vi "Setup_Scan_Range.vi"(7 "Calling VI Ref":refnum<vi>) -> ()   [LabVIEW 2016]
uses:
  <vilib>/Utility/miscctls.llb/LVPointTypeDef.ctl
  Z Scan Standard Action.ctl
panel:
  in  "Exit":bool
  out "Range (µm)":dbl
  out "Step Size (µm)":dbl
  in  "Number of Steps":u16
  out "End Position (µm)":dbl
  out "Start Position (µm)":dbl
  in  "Set End":bool
  in  "Set Start":bool
  # "Copyright (C) 2020 Edward S Allgeyer\n\nRedistribution and use in source and binary forms, with or without\nmodification, are permitted provided that the following conditions\nare met:\n\n1. Redistributions of source code must retain the above copyright\n   notice, this list of conditions and the following disclaimer.\n\n2. Redistributions in binary form must reproduce the above copyright\n   notice, this list of conditions and the following disclaimer in\n   the documentation and/or other materials provided with the\n   distribution.\n\n3. Neither the name of the copyright holder nor the names of its\n   contributors may be used to endorse or promote products derived\n   from this software without specific prior written permission.\n\nTHIS SOFTWARE IS PROVIDED BY THE COPYRIGHT HOLDERS AND CONTRIBUTORS\n\"AS IS\" AND ANY EXPRESS OR IMPLIED WARRANTIES, INCLUDING, BUT NOT\nLIMITED TO, THE IMPLIED WARRANTIES OF MERCHANTABILITY AND FITNESS\nFOR A PARTICULAR PURPOSE ARE DISCLAIMED. IN NO EVENT SHALL THE\nCOPYRIGHT HOLDER OR CONTRIBUTORS BE LIABLE FOR ANY DIRECT, INDIRECT,\nINCIDENTAL, SPECIAL, EXEMPLARY, OR CONSEQUENTIAL DAMAGES (INCLUDING,\nBUT NOT LIMITED TO, PROCUREMENT OF SUBSTITUTE GOODS OR SERVICES;\nLOSS OF USE, DATA, OR PROFITS; OR BUSINESS INTERRUPTION) HOWEVER\nCAUSED AND ON ANY THEORY OF LIABILITY, WHETHER IN CONTRACT, STRICT\nLIABILITY, OR TORT (INCLUDING NEGLIGENCE OR OTHERWISE) ARISING IN\nANY WAY OUT OF THE USE OF THIS SOFTWARE, EVEN IF ADVISED OF THE\nPOSSIBILITY OF SUCH DAMAGE."
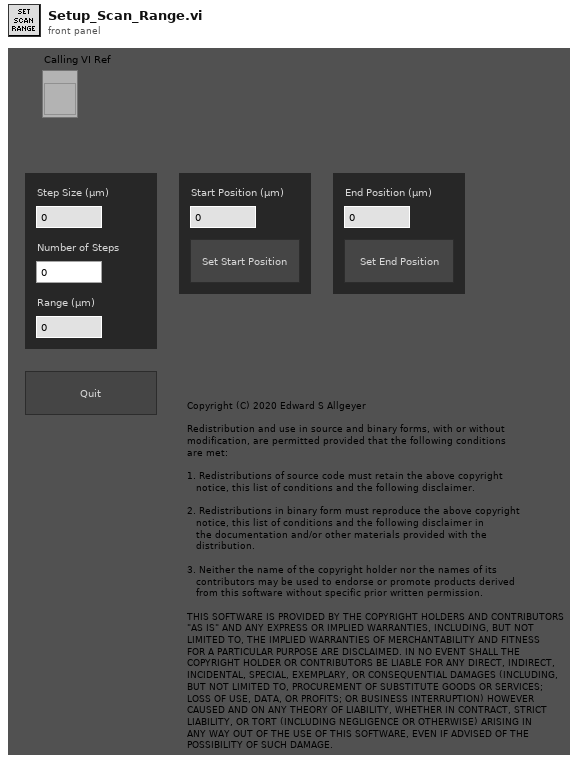
[diagram p1: front panel]
types:
  T1 = enum16{"Always On", "Always Off", "Off While Running"}
  T2 = typedef "LVPointTypeDef.ctl" = cluster{"Horizontal":i16, "Vertical":i16}
  T3 = typedef "Scanning Conversions.ctl" = cluster{"Stage X Axis (Volts/um)":dbl, "Stage Y Axis (Volts/um)":dbl, "Stage Z Axis (Volts/um)":dbl}
  T4 = typedef "Z Scan Standard Action.ctl" = enum16{"Read", "Write"}
  T5 = typedef "Axis Scan Range Parameters.ctl" = cluster{"Start Position (µm)":dbl, "End Position (µm)":dbl, "Step Size (µm)":dbl, "Number of Steps":u16, "Step Direction":bool}
  T6 = typedef "Scan Parameters.ctl" = cluster{"Fast_Ax_Amp_V":dbl, "Fast_Ax_Off_V":dbl, "Slow_Ax_Amp_V":dbl, "Slow_Ax_Off_V ":dbl, "Slow_Ax_Max_V_VperS":dbl, "Slow_Ax1_Del25ns":i32, "Slow_Ax2_Del25ns":i32, "Stage_X_Off_V":dbl, "Stage_Y_Off_V":dbl, "Stage_Z_Off_V":dbl, "Galvo1_Off_V":dbl, "Galvo2_Off_V":dbl, "Last_Scan_Mode":enum16{"XY", "XZ", "YZ", "XYZ"}, "Current_Scan_Mode":enum16{"XY", "XZ", "YZ", "XYZ"}, "Fly_Back_Lines":u16, "Linear_Ramp_End":u32, "Z_Step_I16":i16, "Z_Start_I16":i16, "Laser_States _U32":u32, "590_Voltage_I16":i16, "775_AOM_Volt_I16":i16, "Blanking OFF":bool, "Unused_Axis_I16":i16}
  T7 = typedef "Image Acquisition Parameters.ctl" = cluster{"Scan Type":enum16{"Sample Scanning", "Beam Scanning"}, "Scan Mode":enum16{"XY", "XZ", "YZ", "XYZ"}, "Fast Axis Frequency (Hz)":dbl, "Image Format":u16, "Line Accumulations":u16, "Frames Per Capture":u16, "Frames Accumulations":u16, "Image Dimension (um)":dbl[], "Number of Z Steps":u8, "Z Steps Size (um)":dbl, "Pixel Size (nm)":dbl[]}
  T8 = typedef "LVRectTypeDef.ctl" = cluster{"Left":i16, "Top":i16, "Right":i16, "Bottom":i16}
  T9 = typedef "LVBoundsTypeDef.ctl" = cluster{"Width":u32, "Height":u32}
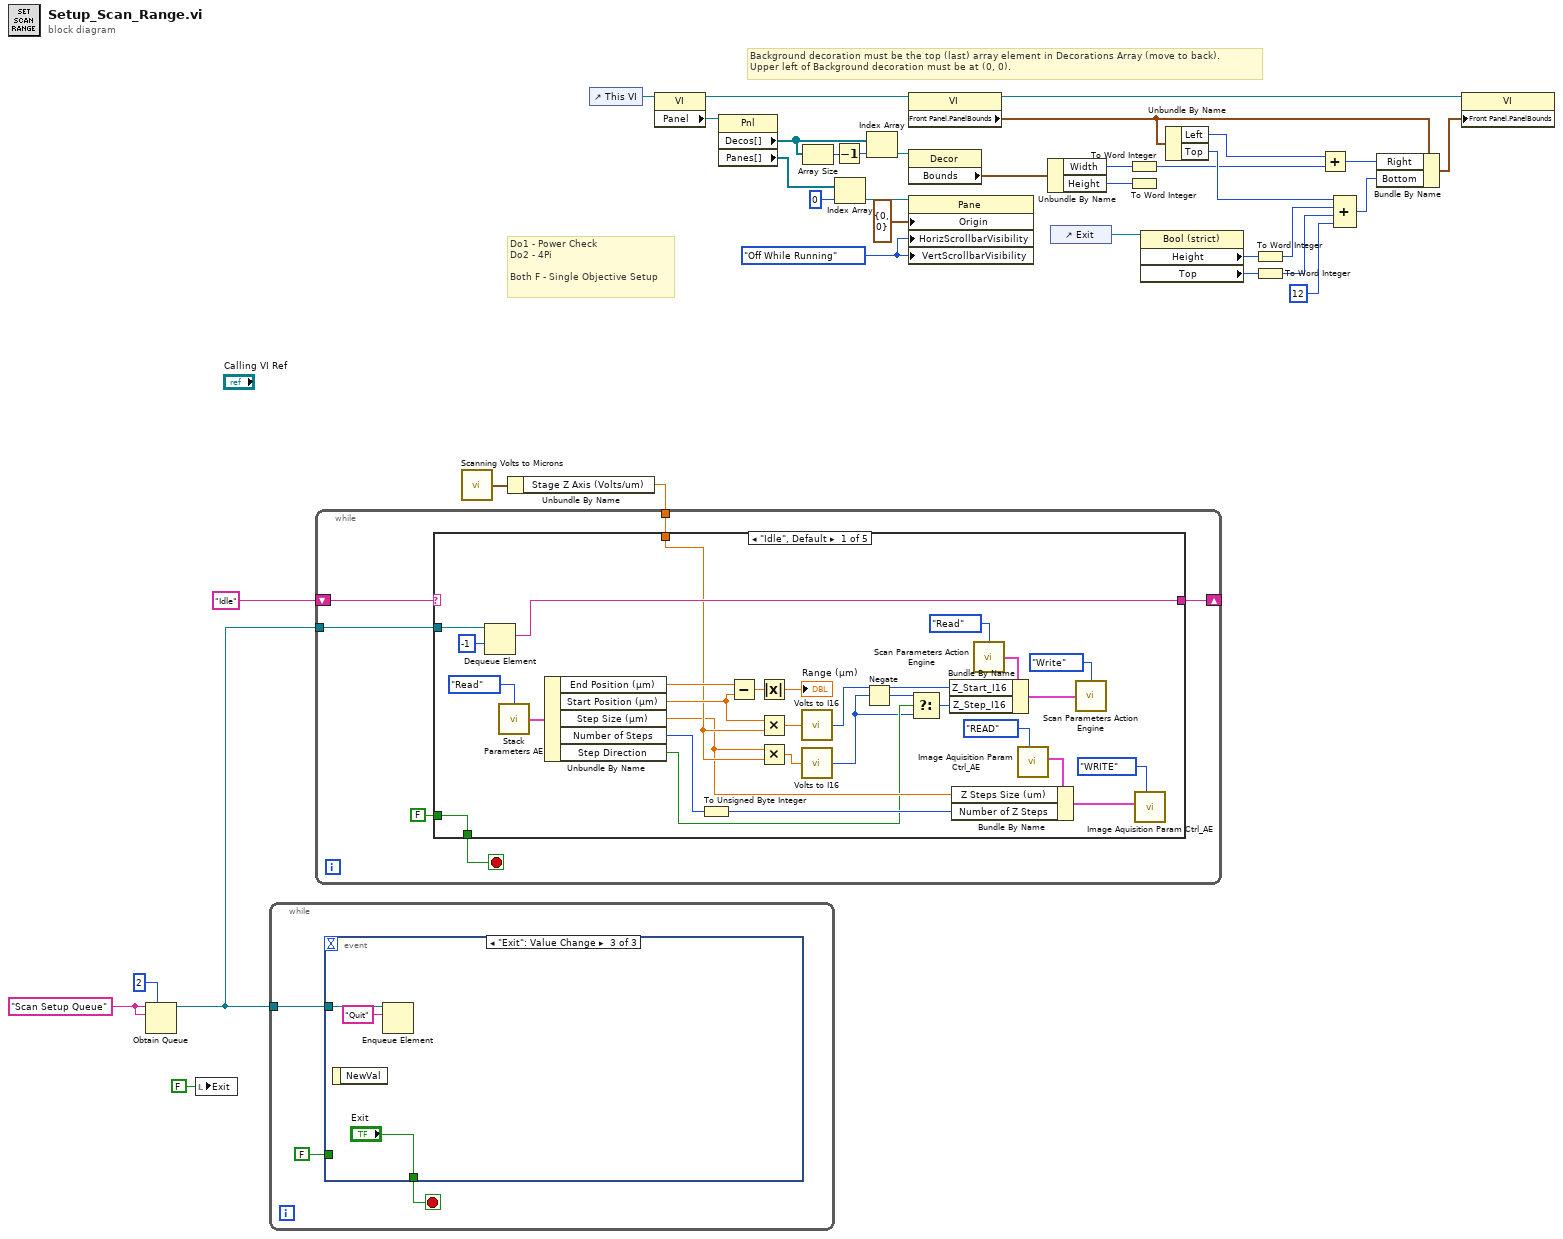
[diagram p0: block diagram]
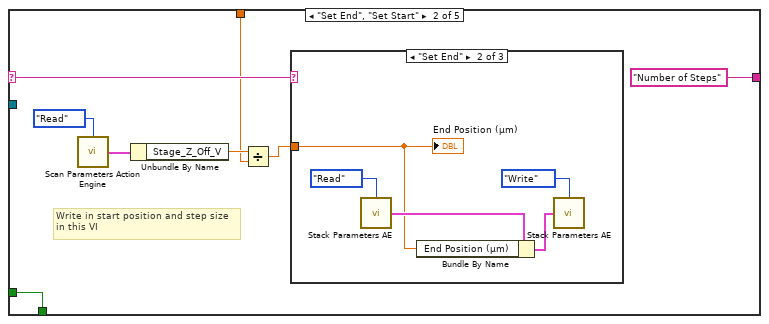
[diagram p2: hidden frame]
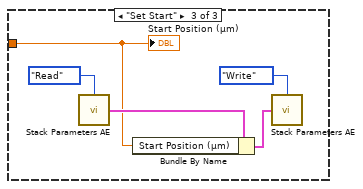
[diagram p4: hidden frame]
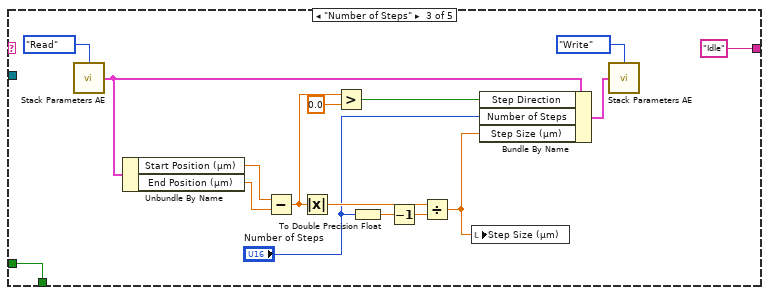
[diagram p5: hidden frame]
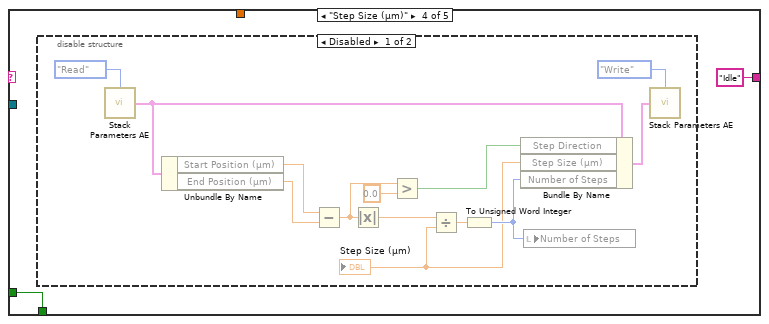
[diagram p6: hidden frame]
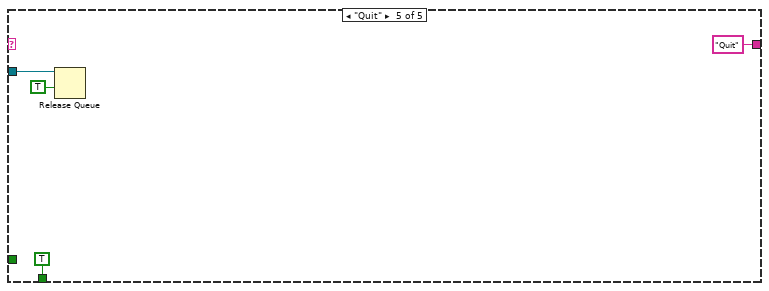
[diagram p8: hidden frame]
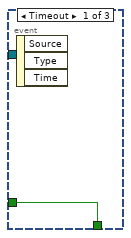
[diagram p9: hidden frame]
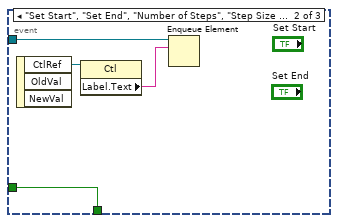
[diagram p10: hidden frame]
diagram:
  w13 = T1."Off While Running" ("Vertical Scrollbar Visibility")
  w35 = "Scan Setup Queue" ("name (unnamed)")
  # "Background decoration must be the top (last) array element in Decorations Array (move to back).\nUpper left of Background decoration must be at (0, 0)."
  # "Do1 - Power Check\nDo2 - 4Pi\n\nBoth F - Single Objective Setup"
  n1 = Obtain Queue(max queue size (-1, unlimited)=2, name (unnamed)=w35, element data type=w35) -> (queue out=w33:refnum<queue>)  [unwired: 2 in, 2 out]
  n2 = local write "Exit"(FALSE ("Exit")) -> ()
  n3 = while {
    tunnel: w33 -> [w37]
    stop <- w39 stop-if-true
    n4 = event shown="[2] \"Exit\": Value Change" {
      selector: _ -> [_ _ _]
      dyn-events: _ -> [_ _ _]
      timeout: _ -> [_ _ _]
      tunnel: [w40 w44 "Exit"] -> w39
      tunnel: FALSE -> [w40 w44 _]
      tunnel: w37 -> [_ w43 w46]
      event Timeout {
        n5 = event-data() -> ()  [unwired: 1 in, 3 out]
      }
      event "Set Start", "Set End", "Number of Steps", "Step Size (µm)": Value Change {
        n6 = event-data() -> ("CtlRef"=w42:refnum<vi>)  [unwired: 1 in, 2 out]
        n7 = property class="Ctl"(reference=w42) -> ("Label.Text"=w41:string)  [unwired: 1 in, 2 out]
        n8 = Enqueue Element(queue=w43, element=w41) -> ()  [unwired: 2 in, 3 out]
      }
      event "Exit": Value Change {
        n9 = event-data() -> ()  [unwired: 1 in, 1 out]
        n10 = Enqueue Element(queue=w46, element="Quit") -> ()  [unwired: 2 in, 3 out]
      }
    }
  }
  n11 = call "Scanning Volts to Microns.vi"() -> ("Scanning Conversions OUT"=w32:T3)
  n12 = Unbundle By Name(w32) -> ("Stage Z Axis (Volts/um)"=w31:dbl)
  n13 = while {
    shift-right: [w51] -> _
    shift-left: "Idle" -> [w53]
    tunnel: w33 -> [w52]
    tunnel: w31 -> [w48]
    stop <- w49 stop-if-true
    n14 = case shown="\"Idle\", Default" w53 {
      selector: w53 -> [_ w88 _ _ _]
      tunnel: w52 -> [w82 _ _ _ w133]
      tunnel: [w80 "Number of Steps" ("name (unnamed)") "Idle" ("name (unnamed)") "Idle" ("name (unnamed)") "Quit" ("name (unnamed)")] -> w51
      tunnel: [w79 w90 w116 w118 TRUE] -> w49
      tunnel: FALSE -> [w79 w90 w116 w118 _]
      tunnel: w48 -> [w72 w85 _ _ _]
      frame "Idle", Default {
        n15 = Dequeue Element(queue=w82, timeout in ms (-1)=-1) -> (element=w80:string)  [unwired: 1 in, 3 out]
        n16 = call "Stack Parameters AE.vi"("Action"=Z_Scan_Standard_Action."Read") -> ("Axis Scan Parameters Out"=w75:T5)  [unwired: 14 in]
        n17 = Unbundle By Name(w75) -> ("End Position (µm)"=w74:dbl, "Start Position (µm)"=w73:dbl, "Step Size (µm)"=w59:dbl, "Number of Steps"=w60:u16, "Step Direction"=w56:bool)
        n18 = To Unsigned Byte Integer(number=w60) -> (unsigned 8bit integer=w58:u8)
        n19 = Subtract(x=w74, y=w73) -> (x-y=w76:dbl)
        n20 = Absolute Value(x=w76) -> (abs(x)=→"Range (µm)":dbl)
        n21 = Multiply(x=w73, y=w72) -> (x*y=w71:dbl)
        n22 = Multiply(x=w59, y=w72) -> (x*y=w70:dbl)
        n23 = call "Volts to I16.vi"("Voltage (V)"=w71) -> ("I16"=w65:i16)  [unwired: 13 in, 1 out]
        n24 = call "Volts to I16.vi"("Voltage (V)"=w70) -> ("I16"=w54:i16)  [unwired: 13 in, 1 out]
        n25 = Negate(x=w54) -> (-x=w55:i16)
        n26 = Select(t=w55, s=w56, f=w54) -> (s? t:f=w57:i16)
        n27 = call "Scan Parameters Action Engine.vi"("Action"=enum16{"Read", "Write"}."Read") -> ("Scan Parameters OUT"=w68:T6)  [unwired: 14 in]
        n28 = Bundle By Name(cluster=w68, "Z_Start_I16"=w65, "Z_Step_I16"=w57) -> (w69:T6)
        n29 = call "Image Aquisition Param Ctrl_AE.vi"("Action"=enum16{"READ", "WRITE"}."READ") -> ("Image Acquisition Parameters Out"=w62:T7)  [unwired: 10 in]
        n30 = Bundle By Name(cluster=w62, "Z Steps Size (um)"=w59, "Number of Z Steps"=w58) -> (w64:T7)
        n31 = call "Scan Parameters Action Engine.vi"("Action"=enum16{"Read", "Write"}."Write", "Scan Parameters IN"=w69) -> ()  [unwired: 13 in, 1 out]
        n32 = call "Image Aquisition Param Ctrl_AE.vi"("Action"=enum16{"READ", "WRITE"}."WRITE", "Image Acquisition Parameters In"=w64) -> ()  [unwired: 9 in, 1 out]
      }
      frame "Set End", "Set Start" {
        # "Write in start position and step size\nin this VI"
        n33 = call "Scan Parameters Action Engine.vi"("Action"=enum16{"Read", "Write"}."Read") -> ("Scan Parameters OUT"=w83:T6)  [unwired: 14 in]
        n34 = Unbundle By Name(w83) -> ("Stage_Z_Off_V"=w86:dbl)
        n35 = Divide(x=w86, y=w85) -> (x/y=w87:dbl)
        n36 = case shown="\"Set End\"" w88 {
          tunnel: w87 -> [_ w92 w96]
          frame Default {
          }
          frame "Set End" {
            n37 = call "Stack Parameters AE.vi"("Action"=Z_Scan_Standard_Action."Read") -> ("Axis Scan Parameters Out"=w93:T5)  [unwired: 14 in]
            n38 = Bundle By Name(cluster=w93, "End Position (µm)"=w92) -> (w91:T5)
            n39 = call "Stack Parameters AE.vi"("Action"=Z_Scan_Standard_Action."Write", "Axis Scan Parameters"=w91) -> ()  [unwired: 13 in, 1 out]
            "End Position (µm)" <- w92
          }
          frame "Set Start" {
            n40 = call "Stack Parameters AE.vi"("Action"=Z_Scan_Standard_Action."Read") -> ("Axis Scan Parameters Out"=w98:T5)  [unwired: 14 in]
            n41 = Bundle By Name(cluster=w98, "Start Position (µm)"=w96) -> (w97:T5)
            n42 = call "Stack Parameters AE.vi"("Action"=Z_Scan_Standard_Action."Write", "Axis Scan Parameters"=w97) -> ()  [unwired: 13 in, 1 out]
            "Start Position (µm)" <- w96
          }
        }
      }
      frame "Number of Steps" {
        n43 = call "Stack Parameters AE.vi"("Action"=Z_Scan_Standard_Action."Read") -> ("Axis Scan Parameters Out"=w106:T5)  [unwired: 14 in]
        n44 = Unbundle By Name(w106) -> ("Start Position (µm)"=w108:dbl, "End Position (µm)"=w107:dbl)
        n45 = Subtract(x=w108, y=w107) -> (x-y=w110:dbl)
        n46 = Absolute Value(x=w110) -> (abs(x)=w112:dbl)
        n47 = Greater?(x=w110, y=0.0) -> (0:w104:bool)
        n48 = To Double Precision Float(number="Number of Steps") -> (double precision float=w111:dbl)
        n49 = Decrement(x=w111) -> (x-1=w101:dbl)
        n50 = Divide(x=w112, y=w101) -> (x/y=w102:dbl)
        n51 = local write "Step Size (µm)"(w102) -> ()
        n52 = Bundle By Name(cluster=w106, "Step Direction"=w104, "Number of Steps"="Number of Steps", "Step Size (µm)"=w102) -> (w105:T5)
        n53 = call "Stack Parameters AE.vi"("Action"=Z_Scan_Standard_Action."Write", "Axis Scan Parameters"=w105) -> ()  [unwired: 13 in, 1 out]
      }
      frame "Step Size (µm)" {
        n54 = disable-structure shown="Disabled" {
          frame Disabled {
            n55 = call "Stack Parameters AE.vi"("Action"=Z_Scan_Standard_Action."Read") -> ("Axis Scan Parameters Out"=w123:T5)  [unwired: 14 in]
            n56 = Unbundle By Name(w123) -> ("Start Position (µm)"=w125:dbl, "End Position (µm)"=w124:dbl)
            n57 = Subtract(x=w125, y=w124) -> (x-y=w126:dbl)
            n58 = Absolute Value(x=w126) -> (abs(x)=w129:dbl)
            n59 = Greater?(x=w126, y=0.0) -> (0:w120:bool)
            n60 = Divide(x=w129, y="Step Size (µm)") -> (x/y=w128:dbl)
            n61 = To Unsigned Word Integer(number=w128) -> (unsigned 16bit integer=w121:u16)
            n62 = Bundle By Name(cluster=w123, "Step Direction"=w120, "Step Size (µm)"="Step Size (µm)", "Number of Steps"=w121) -> (w122:T5)
            n63 = local write "Number of Steps"(w121) -> ()
            n64 = call "Stack Parameters AE.vi"("Action"=Z_Scan_Standard_Action."Write", "Axis Scan Parameters"=w122) -> ()  [unwired: 13 in, 1 out]
          }
          frame Enabled {
          }
        }
      }
      frame "Quit" {
        n65 = Release Queue(queue=w133, force destroy? (F)=TRUE) -> ()  [unwired: 1 in, 3 out]
      }
    }
  }
  n66 = control-ref of="This VI"() -> (w5:refnum<vi>)
  n67 = property class="VI"(reference=w5) -> (reference out=w14:refnum<vi>, "Panel"=w6:refnum<vi>)  [unwired: 1 in, 1 out]
  n68 = property class="Pnl"(reference=w6) -> ("Decos[]"=w4:refnum<vi>[], "Panes[]"=w10:refnum<vi>[])  [unwired: 1 in, 2 out]
  n69 = Array Size(array=w4) -> (size(s)=w2:i32)
  n70 = Decrement(x=w2) -> (x-1=w3:i32)
  n71 = Index Array(array=w10, index=0) -> (element=w9:refnum<vi>)
  n72 = Index Array(array=w4, index=w3) -> (element=w12:refnum<vi>)
  n73 = property class="VI"(reference=w14) -> (reference out=w16:refnum<vi>, "Front Panel.PanelBounds"=w17:T8)  [unwired: 1 in, 1 out]
  n74 = property class="Decor"(reference=w12) -> ("Bounds"=w15:T9)  [unwired: 1 in, 2 out]
  n75 = property class="Pane"(reference=w9, "Origin"=T2 {"Horizontal"=0, "Vertical"=0}, "HorizScrollbarVisibility"=w13, "VertScrollbarVisibility"=w13) -> ()  [unwired: 1 in, 2 out]
  n76 = Unbundle By Name(w15) -> ("Width"=w20:u32, "Height"=w23:u32)
  n77 = control-ref of="Exit"() -> (w7:refnum<vi>)
  n78 = To Word Integer(number=w20) -> (16bit integer=w22:i16)
  n79 = To Word Integer(number=w23) -> ()  [unwired: 1 out]
  n80 = property class="Bool (strict)"(reference=w7) -> ("Height"=w25:u32, "Top"=w26:i32)  [unwired: 1 in, 2 out]
  n81 = Unbundle By Name(w17) -> ("Left"=w19:i16, "Top"=w30:i16)
  n82 = To Word Integer(number=w25) -> (16bit integer=w28:i16)
  n83 = To Word Integer(number=w26) -> (16bit integer=w29:i16)
  n84 = Add(x=w19, y=w22) -> (x+y=w21:i16)
  n85 = Compound Arithmetic op=ADD(w30, w28, w29, i16 12 ("y")) -> (w24:i16)
  n86 = Bundle By Name(cluster=w17, "Right"=w21, "Bottom"=w24) -> (w18:T8)
  n87 = property class="VI"(reference=w16, "Front Panel.PanelBounds"=w18) -> ()  [unwired: 1 in, 2 out]
